vi "Extract Multiplier & Range & Function.vi"(11 "Message hex string":string="Š°°µ³4°³°°\r") -> (3 "Multiplier":dbl)   [LabVIEW 2015, in "VC940.lvlib"]
uses:
  VC940.lvlib
  Controls/Function.ctl
panel:
  out "Function (0..15)":T1
  out "Range (0..6)":i32
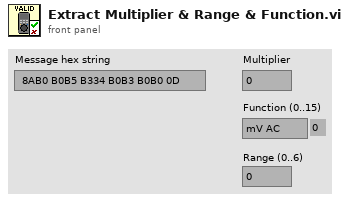
[diagram p1: front panel]
types:
  T1 = typedef "VC940.lvlib/Function.ctl" = enum8{"mV AC", "V DC", "V AC", "mV DC", "Ohm", "nF", "°C", "µA", "mA", "A", "Ohm Fm", "V Diode", "Hz", "°F", "W", "%4-20mA"}
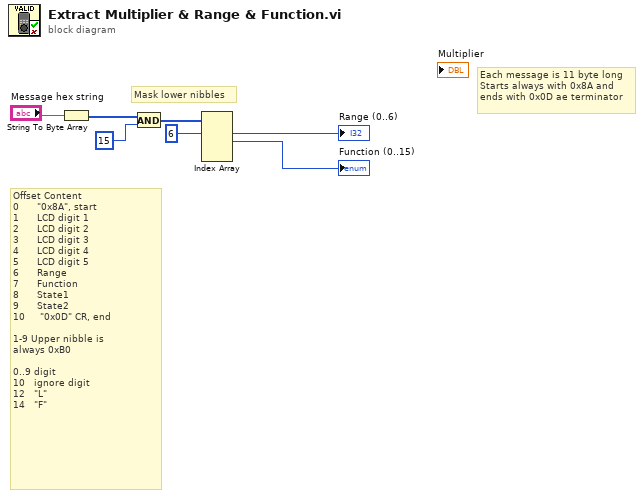
[diagram p0: block diagram]
diagram:
  # "Offset Content\n0      \"0x8A\", start\n1      LCD digit 1\n2      LCD digit 2\n3      LCD digit 3\n4      LCD digit 4\n5      LCD digit 5\n6      Range\n7      Function\n8      State1\n9      State2\n10     \"0x0D\" CR, end\n\n1-9 Upper nibble is\nalways 0xB0\n\n0..9 digit\n10   ignore digit\n12   \"L\"\n14   \"F\""
  # "Mask lower nibbles"
  # "Each message is 11 byte long\nStarts always with 0x8A and\nends with 0x0D ae terminator"
  n1 = String To Byte Array(string="Message hex string") -> (unsigned byte array=w5:u8[])
  n2 = And(x=w5, y=u8 15) -> (x .and. y?=w3:u8[])
  n3 = Index Array(array=w3, index #1=6 ("index")) -> (element #1=→"Range (0..6)":u8, element #2=→"Function (0..15)":u8)  [unwired: 3 in, 2 out]
